vi "Axis_to_string.vi"(0 "Axis":T1) -> (1 "String":string="X Axis", 2 "Reverse Scale":bool, 3 "Index":i32)   [LabVIEW 2010]
uses:
  Axis.ctl
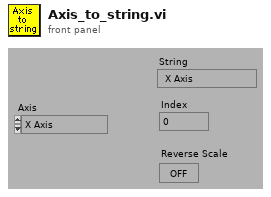
[diagram p1: front panel]
types:
  T1 = typedef "Axis.ctl" = enum16{"X Axis", "X Axis -ve", "Y Axis", "Y Axis -ve", "Z Axis", "Z Axis -ve"}
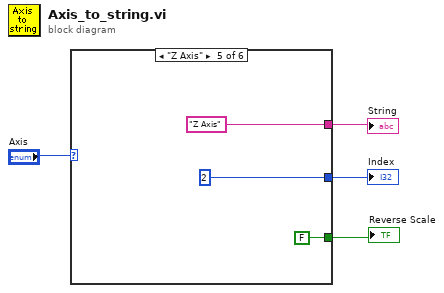
[diagram p0: block diagram]
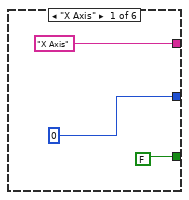
[diagram p2: hidden frame]
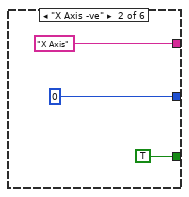
[diagram p3: hidden frame]
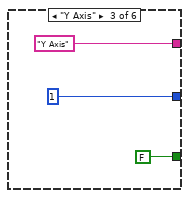
[diagram p4: hidden frame]
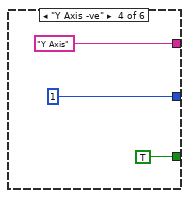
[diagram p5: hidden frame]
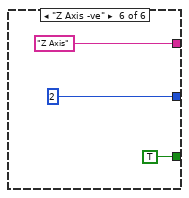
[diagram p6: hidden frame]
diagram:
  n1 = case shown="\"Z Axis\"" "Axis" {
    tunnel: ["X Axis" "X Axis" "Y Axis" "Y Axis" "Z Axis" "Z Axis"] -> w3
    tunnel: [0 0 1 1 2 2] -> w2
    tunnel: [FALSE TRUE FALSE TRUE FALSE TRUE] -> w1
    frame "X Axis" {
    }
    frame "X Axis -ve" {
    }
    frame "Y Axis" {
    }
    frame "Y Axis -ve" {
    }
    frame "Z Axis" {
    }
    frame "Z Axis -ve" {
    }
  }
  "Index" <- w2
  "String" <- w3
  "Reverse Scale" <- w1
